vi "SPD.Save Grid T and Stb.vi"(8 "Error In":errorcluster, 11 "SPD.Stand Ctrl in":T1 {"spdDeviceSession"."hidSPD.Sturtup Values"."HV_bias" format="%#_6p, V"; "spdDeviceSession"."hidSPD.Sturtup Values"."TSet" format="%#_6p, DegC"; "spdDeviceSession"."hidSPD.Controller"."HV_bias" format="%#_6p, V"; "spdDeviceSession"."hidSPD.Controller"."TSet" format="%#_6p, DegC"}) -> (0 "Error Out":errorcluster, 3 "SPD.Stand Ctrl out":T1 {"spdDeviceSession"."hidSPD.Sturtup Values"."HV_bias" format="%#_6p, V"; "spdDeviceSession"."hidSPD.Sturtup Values"."TSet" format="%#_6p, DegC"; "spdDeviceSession"."hidSPD.Controller"."HV_bias" format="%#_6p, V"; "spdDeviceSession"."hidSPD.Controller"."TSet" format="%#_6p, DegC"})   [LabVIEW 2018]
uses:
  typedefs/SPD.Stand Ctrl.ctl
  Instruments/SPD HID Interface/hidSPDLibForLabView/LibVIs/hidSPD Controls/hidSPD Device Session.ctl
  Instruments/SPD HID Interface/hidSPDLibForLabView/LibVIs/hidSPD Controls/hidSPD Controller.ctl
  Instruments/SPD HID Interface/hidSPDLibForLabView/LibVIs/hidSPD Controls/hidSPD SPD Type.ctl
  Instruments/KC705 DevBoard/typedefs/DevB.Session.ctl
  Instruments/KeySight 53230A/typedefs/FreqC.Session.ctl
  Instruments/KeySight 8164B/KeySight 8164B LAN InstrLib/typedefs/KeySight 8164B control.ctl
  Instruments/LeCroy SDA830/typedefs/LeCroy.Session.ctl
  typedefs/SPD.Events.ctl
  ConfigFile/SPD.Config File ctrl.ctl
  <vilib>/Utility/config.llb/Config Data RefNum.ctl
  typedefs/SPD.Meas Result.ctl
  typedefs/SPD.Queues.ctl
  typedefs/SPD.Stand state.ctl
  Instruments/KeySight 8164B/KeySight 8164B LAN InstrLib.lvlib
  <vilib>/Utility/config.llb/NI_LVConfig.lvlib
  Instruments/SPD HID Interface/hidSPDLibForLabView/hidSPDLibForLabView.lvlib
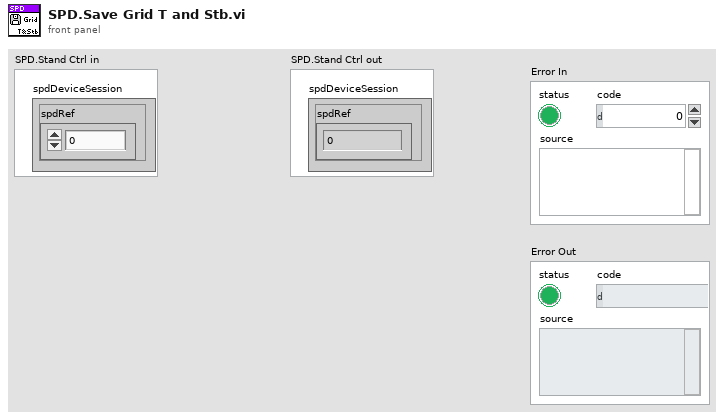
[diagram p1: front panel]
types:
  T1 = typedef "SPD.Stand Ctrl.ctl" = cluster{"spdDeviceSession":T2, "DevBSession":T5, "FreqCSession":T6, "8164BSession":T7, "LeCroySession":T8, "Events":T9, "configFile":T10, "SPD.Result":T12, "SPD.Queues":T13, "Console":refnum<vi>}
  T2 = typedef "hidSPDLibForLabView.lvlib/hidSPD Device Session.ctl" = cluster{"spdRef":u64, "connected":bool, "spdName":string, "hidSPD.Controller":T3, "hidSPD.Sturtup Values":T3, "SPD Type":T4}
  T3 = typedef "hidSPDLibForLabView.lvlib/hidSPD Controller.ctl" = cluster{"TSet":sgl, "HV_bias":sgl, "DDS_stb_code":u16}
  T4 = typedef "hidSPDLibForLabView.lvlib/hidSPD SPD Type.ctl" = enum16{"Free Run", "Gate"}
  T5 = typedef "DevB.Session.ctl" = cluster{"DevBRef":refnum<visa-resource-name>, "connected":bool}
  T6 = typedef "FreqC.Session.ctl" = cluster{"FreqCRef":refnum<visa-resource-name>, "timeout":dbl, "Gate":dbl, "connected":bool}
  T7 = typedef "KeySight 8164B LAN InstrLib.lvlib/KeySight 8164B control.ctl" = cluster{"Connection ID":refnum<k5>, "Connected":bool, "Info":string, "Slots Info":string[]}
  T8 = typedef "LeCroy.Session.ctl" = cluster{"LeCroySession":refnum<visa-resource-name>, "connected":bool}
  T9 = typedef "SPD.Events.ctl" = cluster{"DCRTest":refnum<user-event>, "Stop":refnum<user-event>}
  T10 = typedef "SPD.Config File ctrl.ctl" = cluster{"configFile ref":T11, "configFile path":path, "equipmentFile ref":T11}
  T11 = typedef "NI_LVConfig.lvlib/Config Data RefNum.ctl" = refnum<k1>
  T12 = typedef "SPD.Meas Result.ctl" = cluster{"HV_Bias":dbl[][][], "Stb_code":dbl[], "Temprature":dbl[], "Data":dbl[][][][], "DateTime":string}
  T13 = typedef "SPD.Queues.ctl" = cluster{"state queue":refnum<queue>}
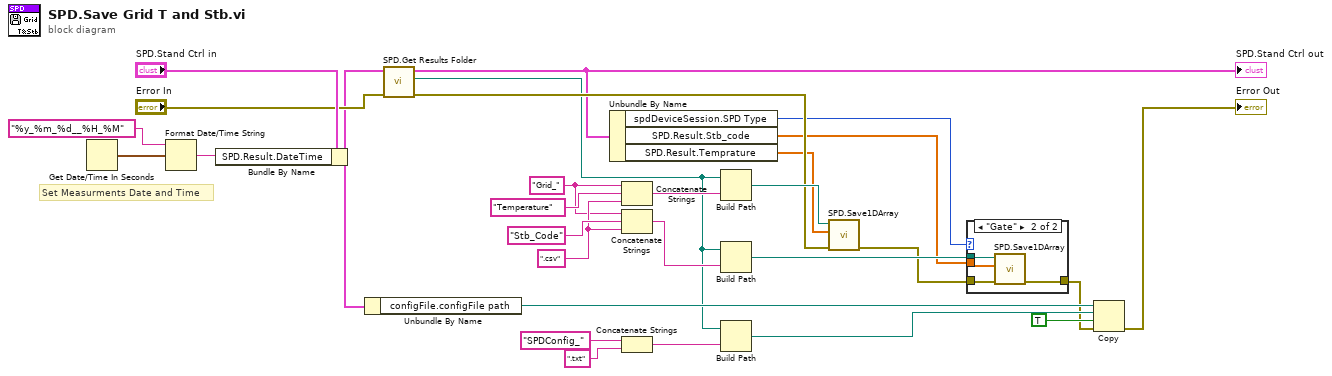
[diagram p0: block diagram]
diagram:
  w18 = ".csv" ("string")
  w17 = "Grid_"
  # "Set Measurments Date and Time"
  n1 = Get Date/Time In Seconds() -> (seconds since 1Jan1904=w16:timestamp)
  n2 = Format Date/Time String(time format string (%c)="%y_%m_%d__%H_%M", seconds (now)=w16) -> (date/time string=w14:string)  [unwired: 1 in]
  n3 = Bundle By Name(cluster="SPD.Stand Ctrl in", "SPD.Result.DateTime"=w14) -> (w11:T1)
  n4 = Unbundle By Name(w11) -> ("configFile.configFile path"=w10:path)
  n5 = call "SPD.Get Results Folder.vi"("Error In"="Error In", "SPD.Stand Ctrl in"=w11) -> ("Error Out"=w24:errorcluster, "Results path"=w9:path, "SPD.Stand Ctrl out"=w20:T1)  [unwired: 7 in]
  "SPD.Stand Ctrl out" <- w20
  n6 = Unbundle By Name(w20) -> ("spdDeviceSession.SPD Type"=w1:T4, "SPD.Result.Stb_code"=w22:dbl[], "SPD.Result.Temprature"=w19:dbl[])
  n7 = Concatenate Strings(w17, "Temperature" ("string"), w18) -> (w28:string)
  n8 = Concatenate Strings(w17, "Stb_Code" ("string"), w18) -> (w26:string)
  n9 = Concatenate Strings("SPDConfig_" ("string"), ".txt" ("string")) -> (w6:string)
  n10 = Build Path(base path=w9, name or relative path=w28) -> (appended path=w25:path)
  n11 = Build Path(base path=w9, name or relative path=w26) -> (appended path=w23:path)
  n12 = Build Path(base path=w9, name or relative path=w6) -> (appended path=w5:path)
  n13 = call "SPD.Save1DArray.vi"("Error In"=w24, "Array"=w19, "File Path"=w25) -> ("Error Out"=w21:errorcluster)  [unwired: 8 in]
  n14 = case shown="\"Gate\"" w1 {
    tunnel: w23 -> [_ w34]
    tunnel: w22 -> [_ w33]
    tunnel: w21 -> [w30 w32]
    tunnel: [w30 w31] -> w3
    frame "Free Run", Default {
    }
    frame "Gate" {
      n15 = call "SPD.Save1DArray.vi"("Error In"=w32, "Array"=w33, "File Path"=w34) -> ("Error Out"=w31:errorcluster)  [unwired: 8 in]
    }
  }
  n16 = Copy(8:w3, 9:TRUE ("overwrite (F)"), 10:w5, 11:w10) -> (0:→"Error Out":errorcluster)  [unwired: 1 in, 2 out]
